vi "Sort_2D_array.vi"(2 "Column index to sort on":i32, 3 "unsorted array":dbl[][](array[numeric]) format="%.2f") -> (0 "Sort Index":i32[](array[numeric]), 1 "sorted array":dbl[][](array[numeric]) format="%.2f")   [LabVIEW 2020]
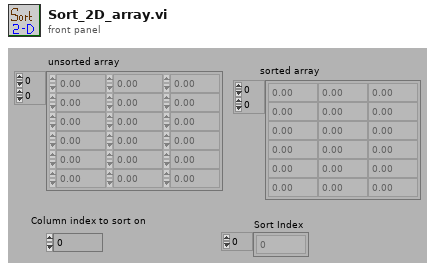
[diagram p1: front panel]
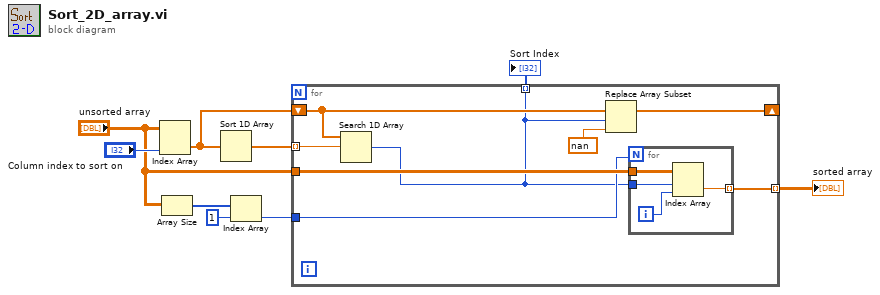
[diagram p0: block diagram]
diagram:
  n1 = Index Array(array="unsorted array", index (col)="Column index to sort on") -> (element=w2:dbl[])  [unwired: 1 in]
  n2 = Array Size(array="unsorted array") -> (size(s)=w6:i32[])
  n3 = Sort 1D Array(array=w2) -> (sorted array=w9:dbl[])
  n4 = Index Array(array=w6, index=1) -> (element=w4:i32)
  n5 = for {
    tunnel: w9 -> [w17] mode=indexing
    tunnel: "unsorted array" -> [w16]
    tunnel: [w15] -> w3 mode=indexing
    tunnel: w4 -> [w14]
    shift-right: [w12] -> _
    shift-left: w2 -> [w13]
    tunnel: [w10] -> w1 mode=indexing
    n6 = Search 1D Array(1D array=w13, element=w17) -> (index of element=w10:i32)  [unwired: 1 in]
    n7 = Replace Array Subset(array=w13, new element=nan ("new element/subarray"), index=w10) -> (w12:dbl[])
    n8 = for {
      N: w14 -> [_]
      tunnel: w16 -> [w21]
      tunnel: w10 -> [w19]
      tunnel: [w18] -> w15 mode=indexing
      i -> [w20]
      n9 = Index Array(array=w21, index (row)=w19, index (col)=w20) -> (element=w18:dbl)
    }
  }
  "sorted array" <- w3
  "Sort Index" <- w1
